vi "SaveBlock.vi"(6 "Registry":T13, 7 "start block":T21, 8 "error in (no error)":errorcluster, 9 "data":T9, 10 "data event config in":T17, 11 "data event":T1) -> (0 "error out":errorcluster, 1 "file complete":bool, 2 "data event config out":T17, 3 "data event out":T1)   [LabVIEW 2017, in "McsaDataEventCreator.lvlib"]
uses:
  <vilib>/addons/InsightCM/Devices/Shared/Mcsa/McsaDataEventCreator/McsaDataEventCreator.lvlib
  <vilib>/addons/InsightCM/Devices/Shared/Common/DVRBuffer/controls/BufferLocation.ctl
  <vilib>/addons/InsightCM/Devices/Shared/Mcsa/McsaDataEventCreator/controls/DataEventConfig.ctl
  <vilib>/addons/InsightCM/Devices/Shared/Mcsa/McsaDataEventCreator/controls/AcqParams.ctl
  <vilib>/addons/InsightCM/Devices/Shared/Common/DataAccumulator/controls/AccumulationSettings.ctl
  <vilib>/addons/InsightCM/Devices/Shared/Common/DataAccumulator/controls/accumulationType.ctl
  <vilib>/addons/PointValueMap/controls/PointMap.ctl
  <vilib>/addons/InsightCM/Devices/Shared/Mcsa/McsaDataEventCreator/controls/DataGroupRegistry.ctl
  <vilib>/addons/InsightCM/Devices/Shared/Mcsa/McsaDataEventCreator/controls/Registry_DataSet.ctl
  <vilib>/addons/InsightCM/Devices/Shared/Mcsa/McsaDataEventCreator/controls/DataSetType.ctl
  <vilib>/addons/InsightCM/Devices/Shared/Common/DataEventCreator/controls/Registry_Trend.ctl
  <vilib>/addons/InsightCM/Devices/Shared/Common/DataFlow/controls/Data.ctl
  <vilib>/addons/InsightCM/Utilities/DataAccessors/controls/wfmSGL_DVR.ctl
  <vilib>/addons/InsightCM/Devices/Shared/Common/DataFlow/controls/Type.ctl
  <vilib>/addons/InsightCM/Devices/Shared/Common/DataEvent/controls/Event.ctl
  <vilib>/addons/InsightCM/MessageBus/Base/controls/DataEvent.ctl
  <vilib>/addons/InsightCM/MessageBus/Base/controls/KeyValuePair.ctl
  <vilib>/addons/InsightCM/Devices/Shared/Common/DataEvent/controls/DataSet.ctl
  <vilib>/addons/InsightCM/MessageBus/Base/controls/DataSetMetadata.ctl
  <vilib>/addons/InsightCM/MessageBus/Base/controls/TrendPoint.ctl
  <vilib>/addons/InsightCM/MessageBus/Base/controls/TrendAlarmUpdate.ctl
  <vilib>/addons/InsightCM/MessageBus/Base/controls/TrendAlarmTransition.ctl
  <vilib>/addons/InsightCM/Devices/Shared/Common/DataAccumulator/controls/DataStoreType.ctl
  <vilib>/addons/InsightCM/Utilities/Analysis/Shared/controls/PulsePositions.ctl
  <vilib>/addons/InsightCM/Devices/Shared/Common/DataAccumulator/DataAccumulator.lvlib
  <vilib>/addons/InsightCM/Utilities/MCSA/McsaUtilities.lvlib
  <vilib>/addons/InsightCM/Devices/Shared/Common/DVRBuffer/DVRBuffer.lvlib
  <vilib>/addons/InsightCM/Utilities/Analysis/Shared/AnalysisHelper.lvlib
  <vilib>/addons/InsightCM/Devices/Shared/Common/DataFlow/DataFlow.lvlib
  <vilib>/addons/PointValueMap/PointValueMap.lvlib
  <vilib>/addons/InsightCM/Devices/Shared/Common/DataEventCreator/DataEventCreator.lvlib
  <vilib>/addons/InsightCM/Devices/Shared/Common/DataEvent/DataEvent.lvlib
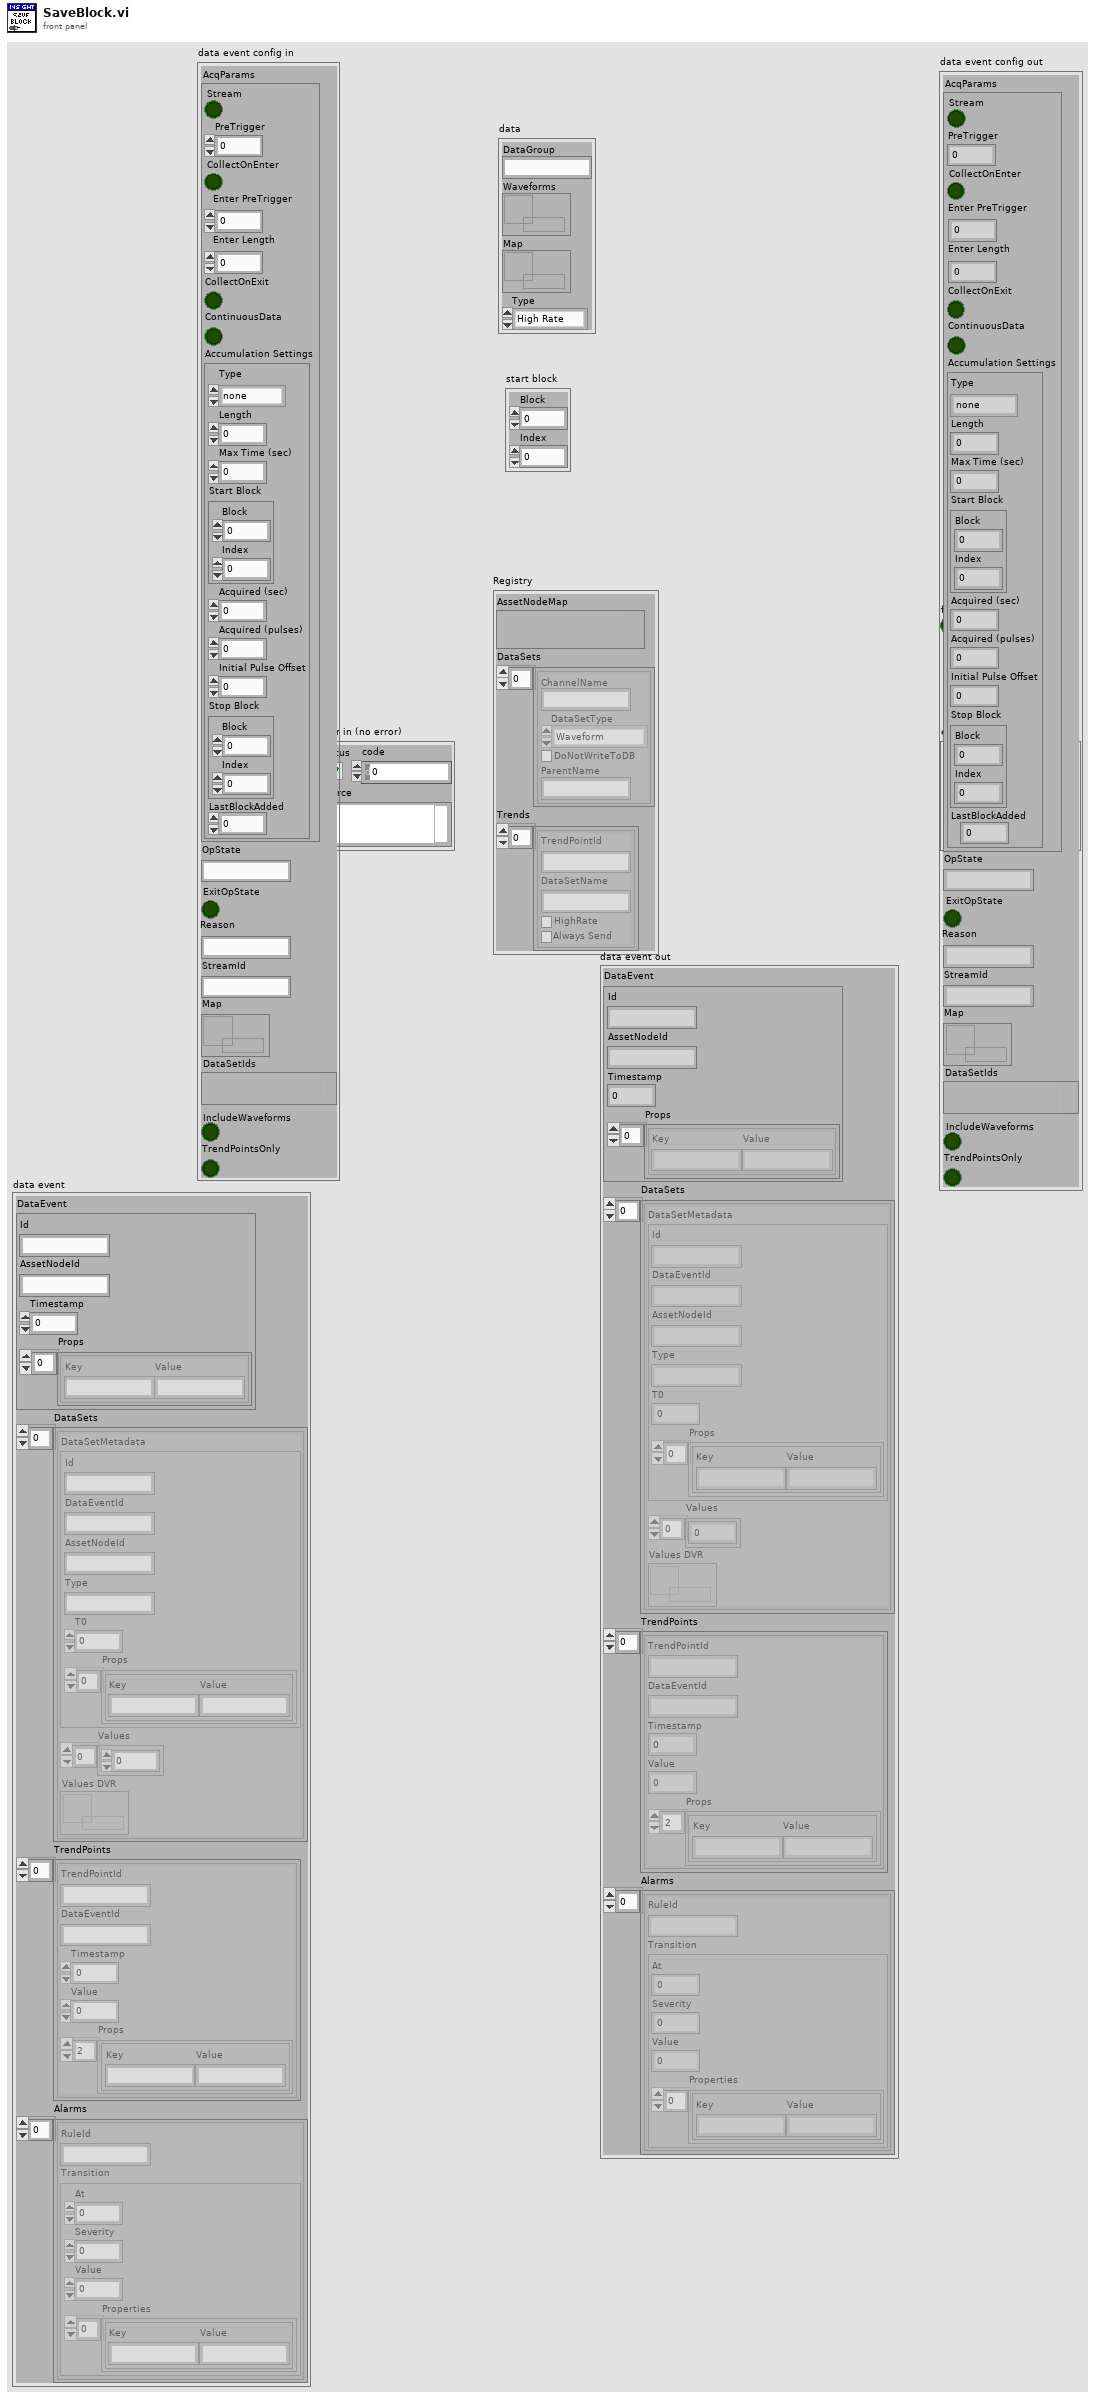
[diagram p1: front panel]
types:
  T1 = typedef "DataEvent.lvlib/Event.ctl" = cluster{"DataEvent":T2, "DataSets":T4[], "TrendPoints":T6[], "Alarms":T7[]}
  T2 = typedef "DataEvent.ctl" = cluster{"Id":string, "AssetNodeId":string, "Timestamp":i64, "Props":T3[]}
  T3 = typedef "KeyValuePair.ctl" = cluster{"Key":string, "Value":string}
  T4 = typedef "DataEvent.lvlib/DataSet.ctl" = cluster{"DataSetMetadata":T5, "Values":sgl[], "Values DVR":refnum<data-value>}
  T5 = typedef "DataSetMetadata.ctl" = cluster{"Id":string, "DataEventId":string, "AssetNodeId":string, "Type":string, "T0":i64, "Props":T3[]}
  T6 = typedef "TrendPoint.ctl" = cluster{"TrendPointId":string, "DataEventId":string, "Timestamp":i64, "Value":dbl, "Props":T3[]}
  T7 = typedef "TrendAlarmUpdate.ctl" = cluster{"RuleId":string, "Transition":T8}
  T8 = typedef "TrendAlarmTransition.ctl" = cluster{"At":i64, "Severity":i32, "Value":dbl, "Properties":T3[]}
  T9 = typedef "DataFlow.lvlib/Data.ctl" = cluster{"DataGroup":string, "Waveforms":T10, "Map":T11, "Type":T12}
  T10 = typedef "wfmSGL_DVR.ctl" = refnum<data-value>
  T11 = typedef "PointValueMap.lvlib/PointMap.ctl" = refnum<data-value>
  T12 = typedef "DataFlow.lvlib/Type.ctl" = enum16{"High Rate", "Low Rate", "Burst Mode"}
  T13 = typedef "McsaDataEventCreator.lvlib/DataGroupRegistry.ctl" = cluster{"AssetNodeMap":variant, "DataSets":T14[], "Trends":T16[]}
  T14 = typedef "McsaDataEventCreator.lvlib/Registry_DataSet.ctl" = cluster{"ChannelName":string, "DataSetType":T15, "DoNotWriteToDB":bool, "ParentName":string}
  T15 = typedef "McsaDataEventCreator.lvlib/DataSetType.ctl" = enum16{"Waveform", "MCSAFFT", "TorqueWFM"}
  T16 = typedef "DataEventCreator.lvlib/Registry_Trend.ctl" = cluster{"TrendPointId":string, "DataSetName":string, "HighRate":bool, "Always Send":bool}
  T17 = typedef "McsaDataEventCreator.lvlib/DataEventConfig.ctl" = cluster{"AcqParams":T18, "OpState":string, "ExitOpState":bool, "Reason":string, "StreamId":string, "Map":T11, "DataSetIds":variant, "IncludeWaveforms":bool, "TrendPointsOnly":bool}
  T18 = typedef "McsaDataEventCreator.lvlib/AcqParams.ctl" = cluster{"Stream":bool, "PreTrigger":i32, "CollectOnEnter":bool, "Enter PreTrigger":i32, "Enter Length":dbl, "CollectOnExit":bool, "ContinuousData":bool, "Accumulation Settings":T19}
  T19 = typedef "DataAccumulator.lvlib/AccumulationSettings.ctl" = cluster{"Type":T20, "Length":dbl, "Max Time (sec)":dbl, "Start Block":T21, "Acquired (sec)":dbl, "Acquired (pulses)":i32, "Initial Pulse Offset":dbl, "Stop Block":T21, "LastBlockAdded":u32}
  T20 = typedef "DataAccumulator.lvlib/accumulationType.ctl" = enum16{"none", "seconds", "revolutions"}
  T21 = typedef "DVRBuffer.lvlib/BufferLocation.ctl" = cluster{"Block":u32, "Index":i32}
  T22 = typedef "DataAccumulator.lvlib/DataStoreType.ctl" = cluster{"Group":string, "waveforms":waveform(sgl)[], "pulse positions array":T23[], "start block":T21}
  T23 = typedef "AnalysisHelper.lvlib/PulsePositions.ctl" = cluster{"Name":string, "Pulse Position Data":dbl[], "Pulses Per Rev":i32}
  T24 = typedef "McsaAnalysisFunctions.lvlib/McsaFFT.ctl" = cluster{"Name":string, "Spectrum":cluster{"f0":dbl, "df":dbl, "magnitude [dB]":dbl[]}, "LineFreq":dbl, "RotorSidebandStep":dbl}
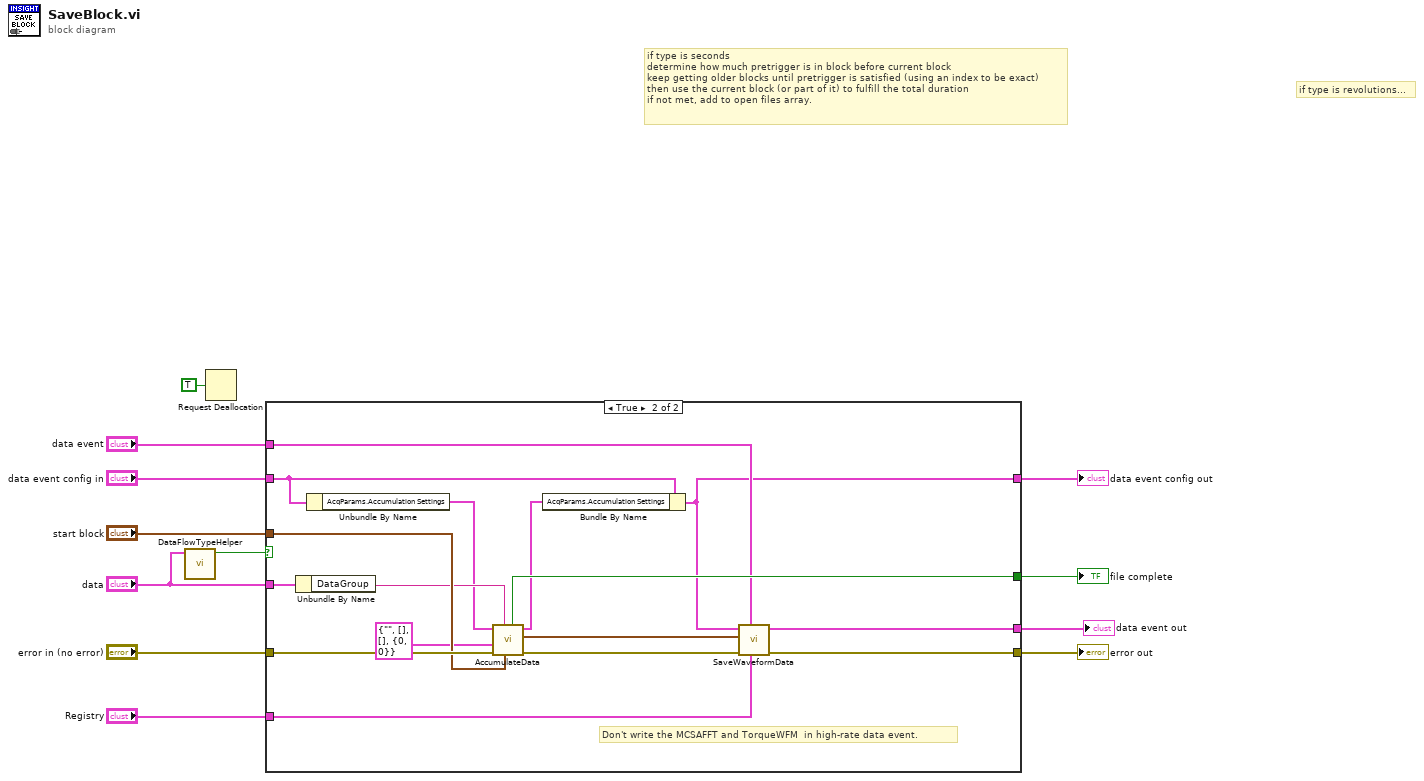
[diagram p0: block diagram]
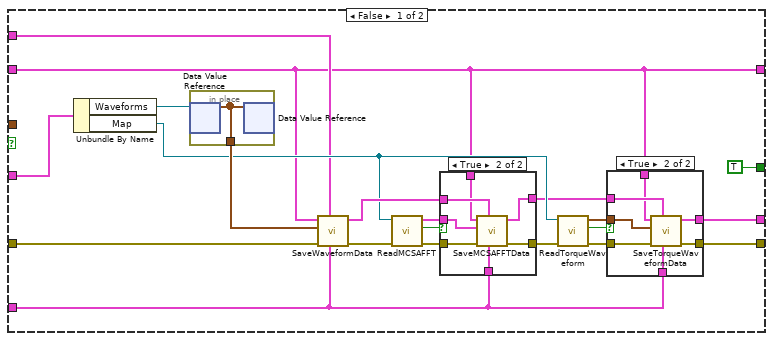
[diagram p2: hidden frame]
diagram:
  # "if type is revolutions..."
  # "if type is seconds\ndetermine how much pretrigger is in block before current block\nkeep getting older blocks until pretrigger is satisfied (using an index to be exact)\nthen use the current block (or part of it) to fulfill the total duration\nif not met, add to open files array."
  n1 = call <vilib>:"DataFlowTypeHelper.vi"("data"="data") -> ("high rate"=w3:bool)  [unwired: 8 in, 2 out]
  n2 = Request Deallocation(TRUE ("flag")) -> ()
  n3 = case shown="True" w3 {
    tunnel: "error in (no error)" -> [w33 w67]
    tunnel: "data event config in" -> [w13 w59]
    tunnel: "Registry" -> [w20 w58]
    tunnel: [w13 w54] -> w9
    tunnel: "start block" -> [_ w66]
    tunnel: [TRUE ("file complete") w64] -> w7
    tunnel: [w21 w57] -> w6
    tunnel: "data" -> [w32 w68]
    tunnel: "data event" -> [w15 w55]
    tunnel: [w14 w53] -> w4
    frame False {
      n4 = Unbundle By Name(w32) -> ("Waveforms"=w31:T10, "Map"=w23:T11)
      n5 = in-place {
        in-place-border: [w52] -> w30
        n6 = in-place-dvr #1(w31) -> (w52:waveform(sgl)[])  [unwired: 1 out]
        n7 = in-place-dvr #1(w52) -> ()  [unwired: 2 out]
      }
      n8 = call <vilib>:"SaveWaveformData.vi"("Registry"=w20, "data event data"=w15, "error in (no error)"=w33, "waveform data"=w30, "data event"=w13) -> ("error out"=w26:errorcluster, "data event data out"=w25:T1)  [unwired: 4 in]
      n9 = call <vilib>:"ReadMCSAFFT.vi"("error in (no error)"=w26, "Map"=w23) -> ("error out"=w28:errorcluster, "found"=w17:bool, "MCSA FFT"=w27:T24)  [unwired: 7 in]
      n10 = case shown="True" w17 {
        tunnel: w28 -> [w44 w51]
        tunnel: w27 -> [_ w50]
        tunnel: w25 -> [w43 w46]
        tunnel: [w44 w49] -> w24
        tunnel: w20 -> [_ w48]
        tunnel: [w43 w47] -> w19
        tunnel: w13 -> [_ w45]
        frame False {
        }
        frame True {
          n11 = call <vilib>:"SaveMCSAFFTData.vi"("Registry"=w48, "data event data"=w46, "error in (no error)"=w51, "MCSA FFT"=w50, "data event"=w45) -> ("error out"=w49:errorcluster, "data event data out"=w47:T1)  [unwired: 5 in]
        }
      }
      n12 = call <vilib>:"ReadTorqueWaveform.vi"("error in (no error)"=w24, "Map"=w23) -> ("error out"=w22:errorcluster, "found"=w16:bool, "Torque Waveform"=w18:waveform(sgl))  [unwired: 7 in]
      n13 = case shown="True" w16 {
        tunnel: w22 -> [w34 w42]
        tunnel: [w34 w41] -> w21
        tunnel: w20 -> [_ w40]
        tunnel: w19 -> [w35 w37]
        tunnel: [w35 w39] -> w14
        tunnel: w18 -> [_ w38]
        tunnel: w13 -> [_ w36]
        frame False {
        }
        frame True {
          n14 = call <vilib>:"SaveTorqueWaveformData.vi"("Registry"=w40, "data event data"=w37, "error in (no error)"=w42, "Torque Waveform"=w38, "data event"=w36) -> ("error out"=w41:errorcluster, "data event data out"=w39:T1)  [unwired: 5 in]
        }
      }
    }
    frame True {
      # "Don't write the MCSAFFT and TorqueWFM  in high-rate data event."
      n15 = Unbundle By Name(w68) -> ("DataGroup"=w65:string)
      n16 = Unbundle By Name(w59) -> ("AcqParams.Accumulation Settings"=w63:T19)
      n17 = call <vilib>:"AccumulateData.vi"("new block"=w66, "data group"=w65, "error in (no error)"=w67, "data in"=T22 {"Group"="", "waveforms"=[], "pulse positions array"=[], "start block"={"Block"=0, "Index"=0}}, "accumulation settings"=w63) -> ("error out"=w60:errorcluster, "waveforms"=w61:waveform(sgl)[], "accumulation settings out"=w62:T19, "accumulation complete"=w64:bool)  [unwired: 1 in, 2 out]
      n18 = Bundle By Name(cluster=w59, "AcqParams.Accumulation Settings"=w62) -> (w54:T17)
      n19 = call <vilib>:"SaveWaveformData.vi"("Registry"=w58, "data event data"=w55, "error in (no error)"=w60, "waveform data"=w61, "data event"=w54) -> ("error out"=w57:errorcluster, "data event data out"=w53:T1)  [unwired: 4 in]
    }
  }
  "error out" <- w6
  "file complete" <- w7
  "data event config out" <- w9
  "data event out" <- w4
